vi "GetFlags.vi"(8 "error in (no error)":errorcluster, 11 "NoFlagImpairPlugin in":refnum<class "NoFlagImpairPlugin.lvclass">) -> (0 "error out":errorcluster, 3 "NoFlagImpairPlugin out":refnum<class "NoFlagImpairPlugin.lvclass">)   [LabVIEW 2017, in "FlagImpairPlugins.lvlib" / "NoFlagImpairPlugin.lvclass"]
uses:
  NoFlagImpairPlugin.lvclass
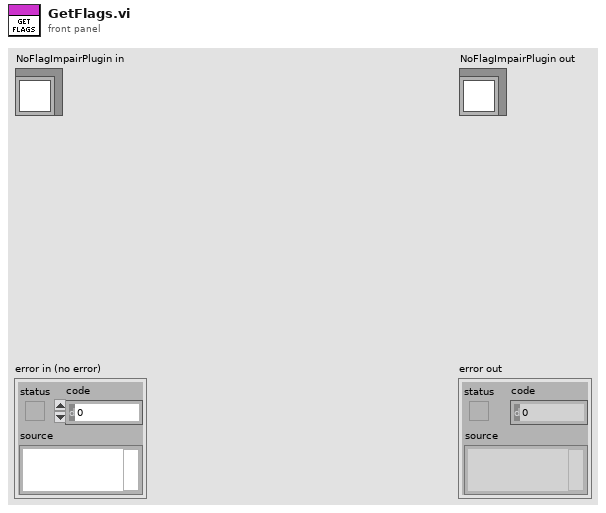
[diagram p1: front panel]
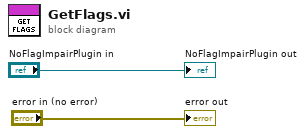
[diagram p0: block diagram]
diagram:
  "error out" <- "error in (no error)"
  "NoFlagImpairPlugin out" <- "NoFlagImpairPlugin in"
